vi "SolvePuzzle.vi"(8 "error in (no error)":errorcluster, 11 "Puzzle in":refnum<class "SudokuBoard.lvclass">) -> (0 "error out":errorcluster, 2 "Solution":i32[][](array[numeric]), 3 "Puzzle out":refnum<class "SudokuBoard.lvclass">)   [LabVIEW 2013, in "SudokuBoard.lvclass"]
uses:
  SudokuBoard.lvclass
  SudukuState/SudokuState.lvclass
  Graph/SearchMethod.ctl
  SudokuBoard.lvclass/SudokuBoard.ctl
  Graph/Graph.lvclass
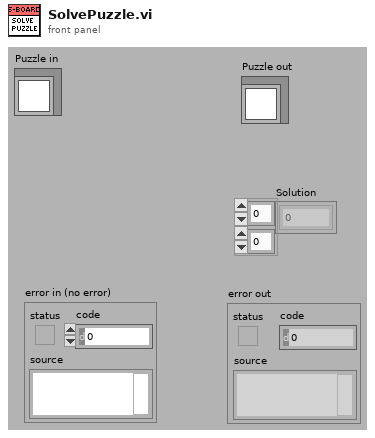
[diagram p1: front panel]
types:
  T1 = typedef "Graph.lvclass/SearchMethod.ctl" = enum16{"Breadth (First)", "Depth (First)", "Best First", "Breadth (Best)", "Depth (Best)"}
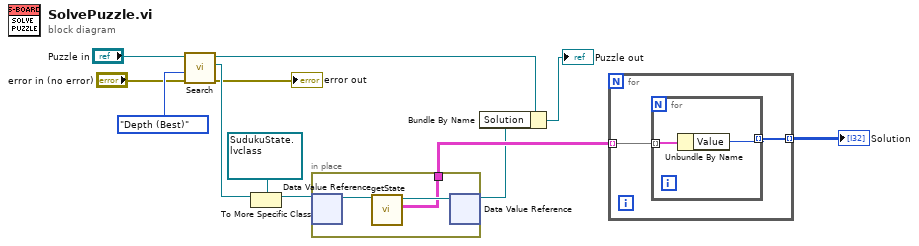
[diagram p0: block diagram]
diagram:
  n1 = call "Search.vi"("error in (no error)"="error in (no error)", "SearchMethod"=SearchMethod."Depth (Best)", "Graph in"="Puzzle in") -> ("error out"=→"error out":errorcluster, "Node"=w10:refnum<data-value>, "Graph out"=w3:refnum<class "SudokuBoard.lvclass">)  [unwired: 5 in, 1 out]
  n2 = To More Specific Class(target class=refnum<data-value> refnum ("data value reference"), reference=w10) -> (specific class reference=w12:refnum<data-value>)  [unwired: 1 in, 1 out]
  n3 = in-place {
    in-place-border: [w13] -> w8
    n4 = in-place-dvr #1(w12) -> (w15:refnum<class "SudokuState.lvclass">)  [unwired: 1 out]
    n5 = call "getState.vi"("SudukuState in"=w15) -> ("State"=w13:cluster{"Value":i32, "Options":i32[]}[][], "SudukuState out"=w14:refnum<class "SudokuState.lvclass">)  [unwired: 8 in, 1 out]
    n6 = in-place-dvr #1(w14) -> (w2:refnum<data-value>)  [unwired: 1 out]
  }
  n7 = Bundle By Name(cluster=w3, "Solution"=w2) -> (→"Puzzle out":refnum<class "SudokuBoard.lvclass">)
  n8 = for {
    tunnel: w8 -> [w17] mode=indexing
    tunnel: [w16] -> w7 mode=indexing
    n9 = for {
      tunnel: w17 -> [w19] mode=indexing
      tunnel: [w18] -> w16 mode=indexing
      n10 = Unbundle By Name(w19) -> ("Value"=w18:i32)
    }
  }
  "Solution" <- w7
